vi "readattribute.vi"() -> ()   [LabVIEW 2020]
uses:
  <vilib>/vision/driver/NI_Vision_Acquisition_Software.lvlib
  <resource>/objmgr/imaqdx.rc
panel:
  out "IsReadable":bool
  out "IsWritable":bool
  out "ValueString":string
  out "error out":errorcluster
  in  "Camera Name":refnum<k21> caption="IMAQdx Session"
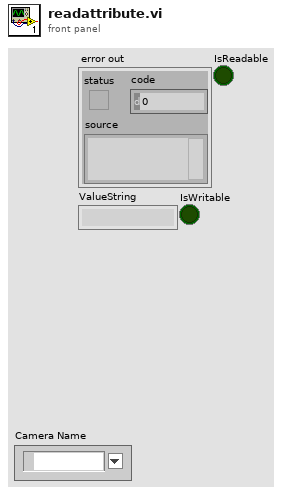
[diagram p1: front panel]
types:
  T1 = typedef "IMAQdx.ctl" = refnum<k21>
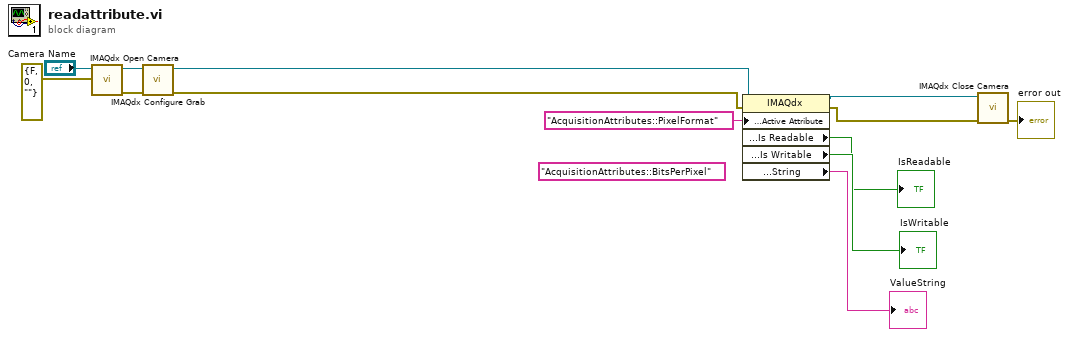
[diagram p0: block diagram]
diagram:
  (unwired) "AcquisitionAttributes::BitsPerPixel" ("ActiveAttribute")
  n1 = call <vilib>:"IMAQdx Open Camera.vi"("error in"=errorcluster {"status"=FALSE, "code"=0, "source"=""}, "Session In"="Camera Name") -> ("error out"=w13:errorcluster, "Session Out"=w12:T1)  [unwired: 1 in, 7 out]
  n2 = call <vilib>:"IMAQdx Configure Grab.vi"("error in"=w13, "Session In"=w12) -> ("error out"=w6:errorcluster, "Session Out"=w8:T1)  [unwired: 1 in, 7 out]
  n3 = property class="IMAQdx"(reference=w8, error in=w6, "Camera Attributes:Active Attribute"="AcquisitionAttributes::PixelFormat" ("ActiveAttribute")) -> (reference out=w7:T1, error out=w5:errorcluster, "Camera Attributes:Is Readable"=→"IsReadable":bool, "Camera Attributes:Is Writable"=→"IsWritable":bool, "Camera Attributes:Value:String"=→"ValueString":string)
  n4 = call <vilib>:"IMAQdx Close Camera.vi"("error in"=w5, "Session In"=w7) -> ("error out"=→"error out":errorcluster)  [unwired: 9 out]
